vi "Handle Error.vi"(8 "error in (no error)":errorcluster, 11 "Core in":refnum<class "Core.lvclass">) -> (0 "error out":errorcluster, 2 "stop actor?":bool=TRUE, 3 "Core out":refnum<class "Core.lvclass">)   [LabVIEW 2019, in "Core.lvlib" / "Core.lvclass"]
doc: "(<B>Filename</B>: Actor Framework.lvlib:Actor.lvclass:Handle Error.vi)\n\nDefines how the actor handles an error that occurred while processing a message. By default, this method does nothing except stop the actor."
uses:
  Core.lvclass
  ModuleAbstract/ModuleAbstract.lvclass
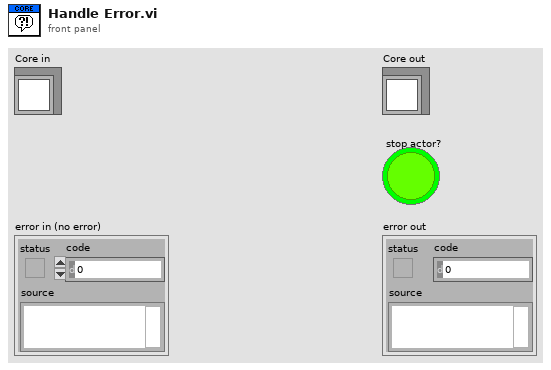
[diagram p1: front panel]
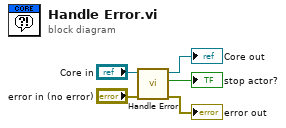
[diagram p0: block diagram]
diagram:
  n1 = call-parent "Handle Error.vi"("error in (no error)"="error in (no error)", "ModuleAbstract in"="Core in") -> ("error out"=→"error out":errorcluster, "stop actor?"=→"stop actor?":bool, "ModuleAbstract out"=→"Core out":refnum<class "Core.lvclass">)  [unwired: 7 in]
